vi "Calibration_Analysis.vi"(2 "Root Name":string[](array[string]), 3 "New Calib Filenames":path[](array[path]), 4 "Instrument type":T1=enum."Hot wire", 5 "Clear Calib History":bool) -> (0 "Error String":string, 1 "Max % Error":dbl format="%.2f")   [LabVIEW 2022 SP3]
uses:
  Controls/Cal_Inst_type.ctl
  Globals/Preference_global.vi
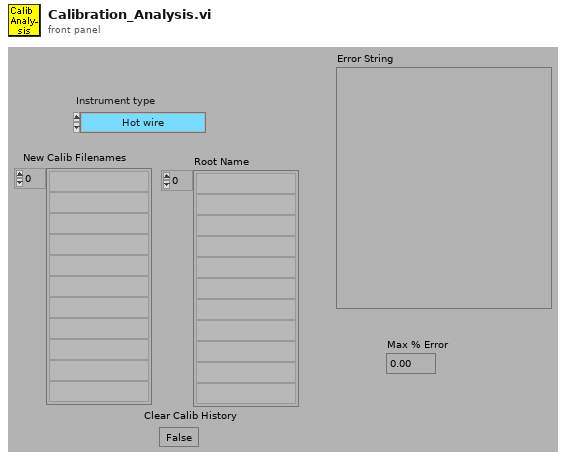
[diagram p1: front panel]
types:
  T1 = typedef "Cal_Inst_type.ctl" = enum16{"Propeller anemometer", "Pressure Transducer", "Hot wire", "Cross wire velocity", "Cross wire angle", "Generic Linear", "Generic Polynomial", "Poly Fit Special", "Fast FID", "Thermocouple", "Cold wire", "Pulsed Wire"}
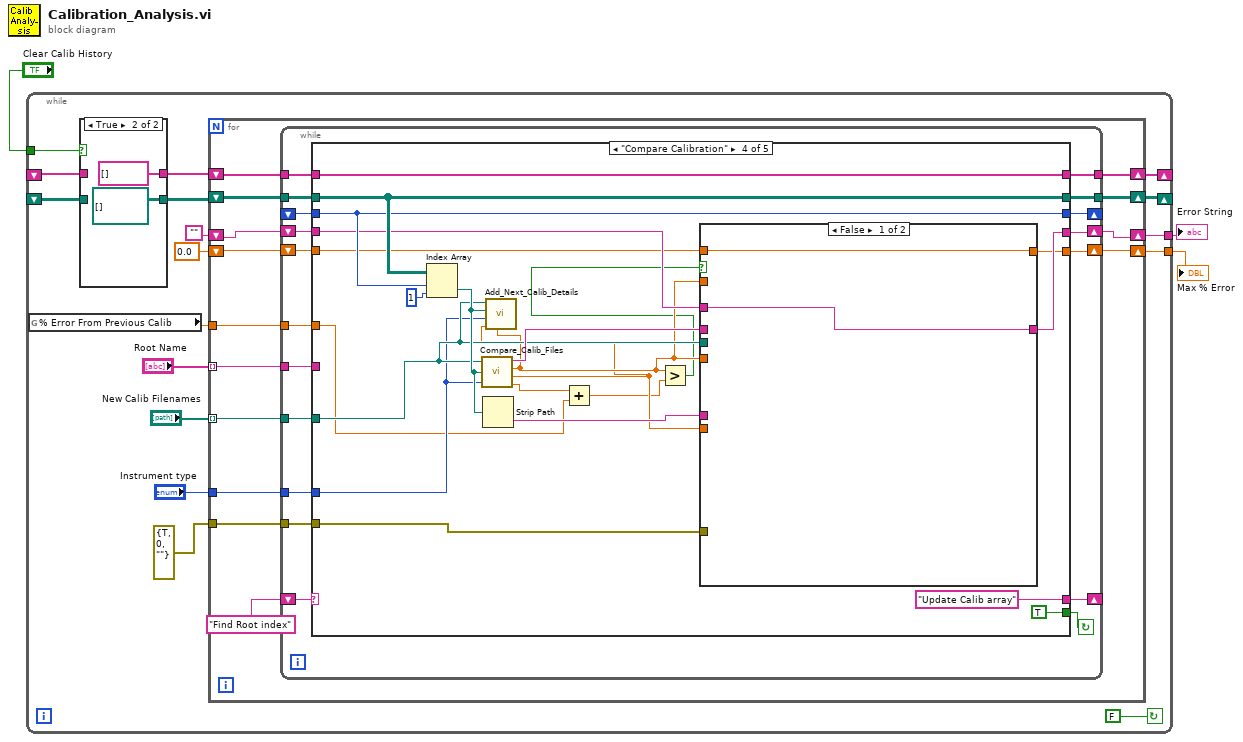
[diagram p0: block diagram]
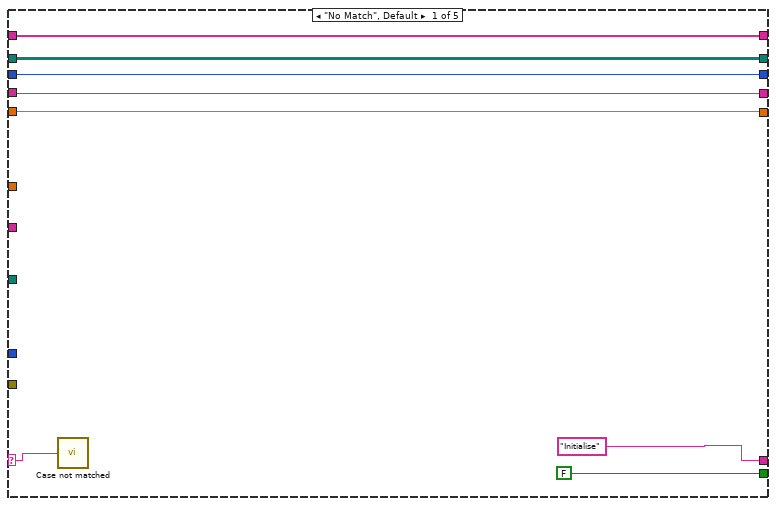
[diagram p3: hidden frame]
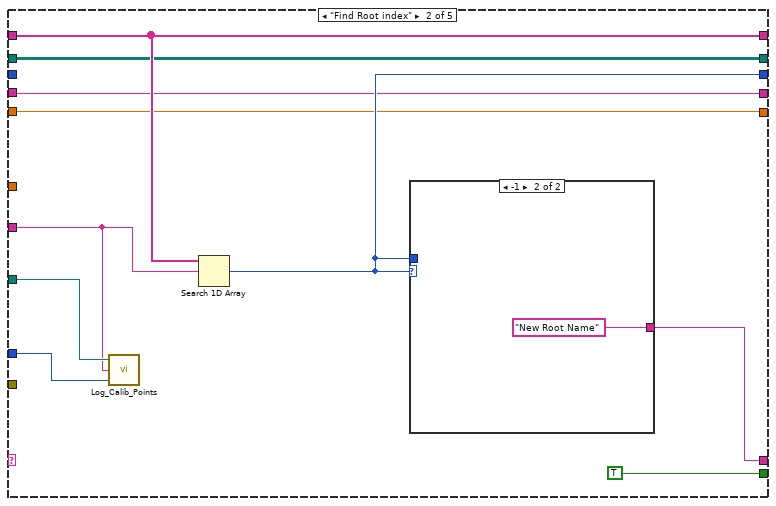
[diagram p4: hidden frame]
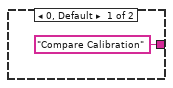
[diagram p5: hidden frame]
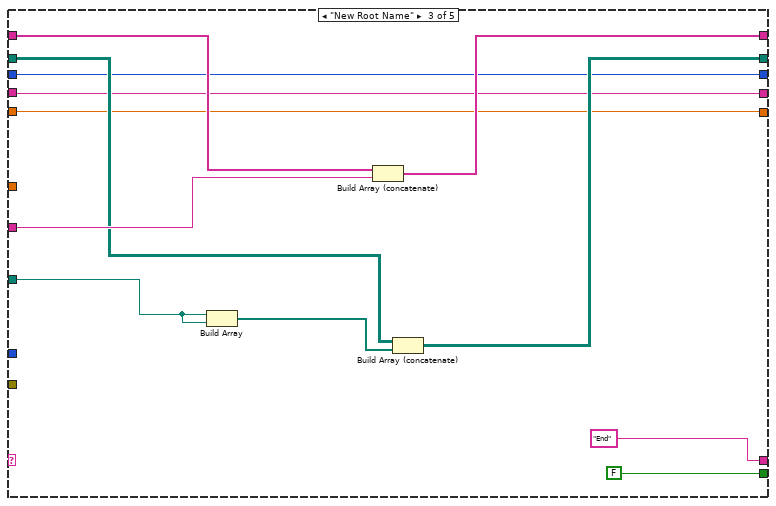
[diagram p6: hidden frame]
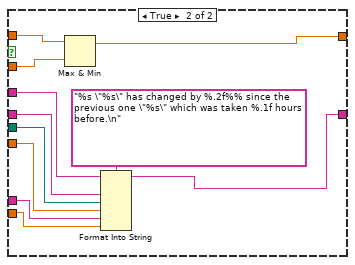
[diagram p7: hidden frame]
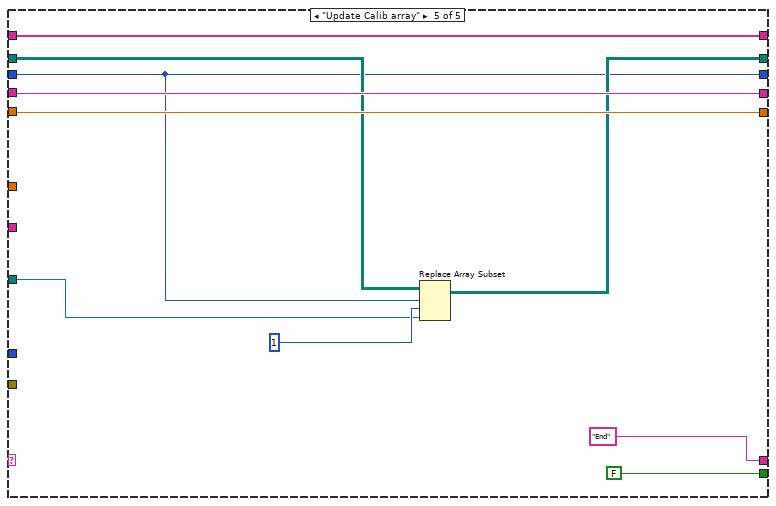
[diagram p8: hidden frame]
diagram:
  n1 = while {
    tunnel: "Clear Calib History" -> [w10]
    tunnel: [w12] -> w2
    tunnel: [w13] -> w3
    shift-left: _ -> [w6]
    shift-right: [w19] -> _
    shift-left: _ -> [w9]
    shift-right: [w20] -> _
    stop <- FALSE continue-if-true
    n2 = global read "Preference_global.vi" "% Error From Previous Calib"() -> (w5:dbl)
    n3 = case shown="True" w10 {
      tunnel: w9 -> [w22 _]
      tunnel: [w22 string[] []] -> w8
      tunnel: [w21 path[][] []] -> w7
      tunnel: w6 -> [w21 _]
      frame False {
      }
      frame True {
      }
    }
    n4 = for {
      shift-right: [w37] -> w20
      shift-left: w8 -> [w36]
      shift-right: [w35] -> w19
      shift-left: w7 -> [w34]
      tunnel: "Root Name" -> [w33] mode=indexing
      tunnel: "New Calib Filenames" -> [w32] mode=indexing
      tunnel: "Instrument type" -> [w31]
      tunnel: errorcluster {"status"=TRUE, "code"=0, "source"=""} ("error in (no error)") -> [w30]
      shift-right: [w28] -> w13
      shift-left: "" -> [w29]
      shift-right: [w26] -> w12
      shift-left: 0.0 -> [w27]
      tunnel: w5 -> [w25]
      n5 = while {
        tunnel: w25 -> [w39]
        shift-left: w27 -> [w40]
        shift-right: [w41] -> w26
        shift-left: w29 -> [w43]
        shift-right: [w42] -> w28
        tunnel: w30 -> [w44]
        tunnel: w31 -> [w45]
        tunnel: w32 -> [w46]
        tunnel: w33 -> [w48]
        shift-left: _ -> [w47]
        shift-right: [w49] -> _
        tunnel: w34 -> [w50]
        tunnel: [w51] -> w35
        tunnel: w36 -> [w52]
        tunnel: [w53] -> w37
        shift-left: "Find Root index" -> [w54]
        shift-right: [w55] -> _
        stop <- w56 continue-if-true
        n6 = case shown="\"Compare Calibration\"" w54 {
          selector: w54 -> [w57 _ _ _ _]
          tunnel: [FALSE TRUE FALSE TRUE FALSE] -> w56
          tunnel: ["Initialise" w72 "End" "Update Calib array" "End"] -> w55
          tunnel: [w62 w73 w85 w110 w133] -> w53
          tunnel: w52 -> [w62 w73 w87 w110 w133]
          tunnel: [w61 w70 w82 w105 w128] -> w51
          tunnel: w50 -> [w61 w70 w83 w105 w126]
          tunnel: [w60 w71 w81 w104 w125] -> w49
          tunnel: w48 -> [_ w66 w86 _ _]
          tunnel: w47 -> [w60 _ w81 w104 w125]
          tunnel: w46 -> [_ w67 w84 w96 w124]
          tunnel: w45 -> [_ w65 _ w95 _]
          tunnel: w44 -> [_ _ _ w107 _]
          tunnel: w43 -> [w59 w69 w78 w102 w132]
          tunnel: [w59 w69 w78 w103 w132] -> w42
          tunnel: [w58 w68 w77 w100 w131] -> w41
          tunnel: w40 -> [w58 w68 w77 w99 w131]
          tunnel: w39 -> [_ _ _ w91 _]
          frame "No Match", Default {
            n7 = call "Case not matched.vi"("Case Name not Matched"=w57) -> ()
          }
          frame "Find Root index" {
            n8 = call "Log_Calib_Points.vi"("Instrument type"=w65, "Root name"=w66, "Calib file"=w67) -> ()  [unwired: 3 out]
            n9 = Search 1D Array(1D array=w73, element=w66) -> (index of element=w71:i32)  [unwired: 1 out]
            n10 = case shown="-1" w71 {
              tunnel: ["Compare Calibration" "New Root Name"] -> w72
              tunnel: w71 -> [_ _]
              frame 0, Default {
              }
              frame -1 {
              }
            }
          }
          frame "New Root Name" {
            n11 = Build Array(w84, w84) -> (w88:path[])
            n12 = Build Array (concatenate)(w87, w86) -> (w85:string[])
            n13 = Build Array (concatenate)(w83, w88) -> (w82:path[][])
          }
          frame "Compare Calibration" {
            n14 = Index Array(array=w105, index (row)=w104, index (col)=1 ("Index")) -> (element=w97:path)
            n15 = call "Compare_Calib_Files.vi"("Calib file New"=w96, "Calib file Orig"=w97, "Instrument type"=w95) -> ("Calib name"=w106:string, "% Change"=w94:dbl, "Calib Time Separation (Hours)"=w93:dbl, "Temperature Change"=w92:dbl)
            n16 = Strip Path(path=w97) -> (name=w98:string)  [unwired: 1 out]
            n17 = call "Add_Next_Calib_Details.vi"("% Change"=w94, "Hours between calibrations"=w93, "Instrument type"=w95, "Calib file Orig"=w97, "Calib file New"=w96) -> ()  [unwired: 2 out]
            n18 = Add(x=w92, y=w91) -> (x+y=w90:dbl)
            n19 = Greater?(x=w94, y=w90) -> (0:w89:bool)
            n20 = case shown="False" w89 {
              tunnel: w107 -> [_ _]
              tunnel: w93 -> [_ w117]
              tunnel: w94 -> [_ w120]
              tunnel: w106 -> [_ w122]
              tunnel: w96 -> [_ w121]
              tunnel: w102 -> [w112 w119]
              tunnel: [w112 w118] -> w103
              tunnel: w94 -> [_ w115]
              tunnel: [w111 w113] -> w100
              tunnel: w99 -> [w111 w114]
              tunnel: w98 -> [_ w116]
              frame False {
              }
              frame True {
                n21 = Max & Min(x=w114, y=w115) -> (max(x,y)=w113:dbl)  [unwired: 1 out]
                n22 = Format Into String(format string="%s \"%s\" has changed by %.2f%% since the previous one \"%s\" which was taken %.1f hours before.\n" ("Format String"), initial string=w119, w122, w121, w120, w116, w117) -> (resulting string=w118:string)  [unwired: 1 in, 1 out]
              }
            }
          }
          frame "Update Calib array" {
            n23 = Replace Array Subset(array=w126, new element=w124, index (row)=w125, index (col)=1 ("Index")) -> (w128:path[][])
          }
        }
      }
    }
  }
  "Error String" <- w3
  "Max % Error" <- w2
